vi "Custom Types in Meta Data.vi"() -> ()   [LabVIEW 2016, in "Tree Manager.lvclass"]
uses:
  Tree Manager.lvclass
  Data Types/Bool/Bool.lvclass/Bool.ctl
  Data Types/Bool/To Bool Tree Data.vi
  Data Types/Bool/From Bool Tree Data.vi
  <vilib>/Utility/error.llb/Clear Errors.vi
  Data Types/Bool/Bool.lvclass
  C:/Users/plkruczp/Google Drive/MyCode/Modules/Tree/Tree Data/Tree Data.lvclass
  API/Get Attribute Tree Data.vi
  API/Set Attribute Tree Data.vi
  Tree Data/Tree Data.lvclass
  Data Types/Int/From Integer Tree Data.vi
  Data Types/Int/Integer.lvclass
panel:
  out "Extracted From Meta Data":errorcluster
  out "Error Status":bool
  in  "Saved Error Info":errorcluster
  in  "Tree":string(tree)
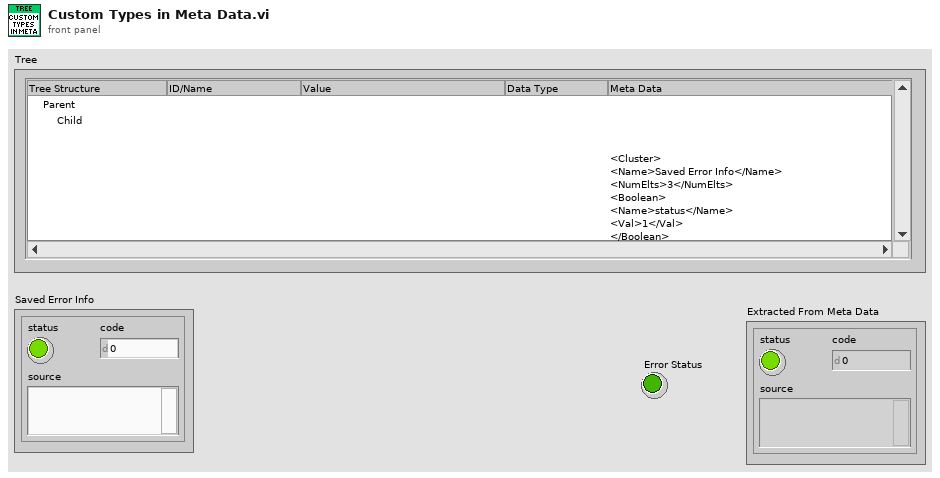
[diagram p1: front panel]
types:
  T1 = typedef "Tree Manager.lvclass/Session Handle.ctl" = refnum<data-value>
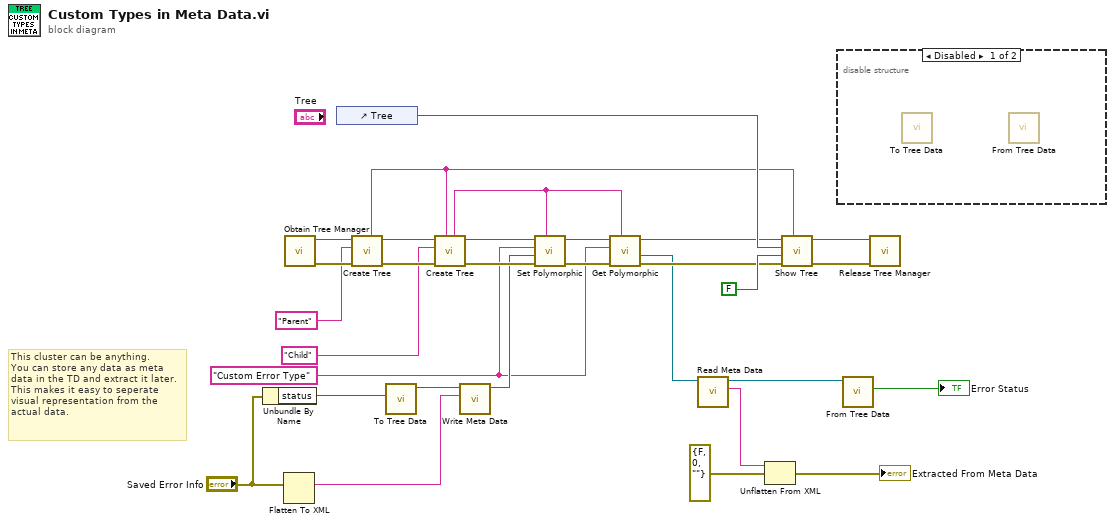
[diagram p0: block diagram]
diagram:
  w11 = "Custom Error Type" ("Name")
  # "This cluster can be anything.\nYou can store any data as meta\ndata in the TD and extract it later.\nThis makes it easy to seperate\nvisual representation from the \nactual data."
  n1 = Unbundle By Name("Saved Error Info") -> ("status"=w7:bool)
  n2 = Flatten To XML(anything="Saved Error Info") -> (xml string=w5:string)
  n3 = call "Obtain Tree Manager.vi"() -> ("Error Out"=w29:errorcluster, "Tree Manager"=w30:T1)  [unwired: 10 in]
  n4 = control-ref of="Tree"() -> (w24:refnum<vi>)
  n5 = call "Create Tree.vi"("Error In"=w29, "Name"="Parent", "Tree Manager"=w30) -> ("Error Out"=w27:errorcluster, "Tree Manager"=w28:T1, "Unique ID"=w17:string)  [unwired: 6 in]
  n6 = call-poly "To Tree Data.vi"("Boolean"=w7) -> ("Bool Tree Data"=w18:refnum<class "Bool.lvclass">)  [unwired: 10 in]
  n7 = call "Create Tree.vi"("Parent ID (empty)"=w17, "Error In"=w27, "Name"="Child", "Tree Manager"=w28) -> ("Error Out"=w22:errorcluster, "Tree Manager"=w23:T1, "Unique ID"=w10:string)  [unwired: 5 in]
  n8 = call "Write Meta Data.vi"("Meta Data"=w5, "Tree Data In"=w18) -> ("Tree Data Out"=w21:refnum<class "Bool.lvclass">)  [unwired: 9 in]
  n9 = call-poly "Set Polymorphic.vi"("Tree ID"=w10, "Error In"=w22, "Attribute Value"=w21, "Attribute Name"=w11, "Tree Manager"=w23) -> ("Error Out"=w14:errorcluster, "Tree Manager"=w15:T1)  [unwired: 4 in, 1 out]
  n10 = call-poly "Get Polymorphic.vi"("Tree ID"=w10, "Error In"=w14, "Attribute Name"=w11, "Tree Manager"=w15) -> ("Error Out"=w12:errorcluster, "Attribute Value"=w9:refnum<class "Tree Data.lvclass">, "Tree Manager"=w13:T1)  [unwired: 4 in, 1 out]
  n11 = call "Read Meta Data.vi"("Tree Data In"=w9) -> ("Meta Data"=w3:string, "Tree Data Out"=w8:refnum<class "Tree Data.lvclass">)  [unwired: 9 in]
  n12 = Unflatten From XML(xml string=w3, type=errorcluster {"status"=FALSE, "code"=0, "source"=""} ("error in (no error)")) -> (value=→"Extracted From Meta Data":errorcluster)  [unwired: 1 in, 1 out]
  n13 = call "Show Tree.vi"("Root ID"=w17, "Error In"=w12, "Show IDs (True)"=FALSE, "Tree Ref"=w24, "Tree Manager"=w13) -> ("Error Out"=w19:errorcluster, "Tree Manager"=w20:T1)  [unwired: 5 in]
  n14 = disable-structure shown="Disabled" {
    frame Disabled {
      n15 = call-poly "To Tree Data.vi"() -> ()  [unwired: 11 in, 1 out]
      n16 = call-poly "From Tree Data.vi"() -> ()  [unwired: 11 in, 1 out]
    }
    frame Enabled {
    }
  }
  n17 = call-poly "From Tree Data.vi"("Tree Data"=w8) -> ("Boolean"=→"Error Status":bool)  [unwired: 10 in]
  n18 = call "Release Tree Manager.vi"("Error In"=w19, "Tree Manager"=w20) -> ()  [unwired: 9 in, 1 out]
